vi "SetInstrument type.vi"(0 "object in":refnum<class "KE2410.lvclass">, 1 "Instrument type":enum16{""}(ring), 5 "error in (no error)":errorcluster) -> (14 "object out":refnum<class "KE2410.lvclass">, 19 "error out":errorcluster)   [LabVIEW 2013, in "KE2410.lvclass"]
uses:
  KE2410.lvclass
  KE2410.lvclass/KE2410.ctl
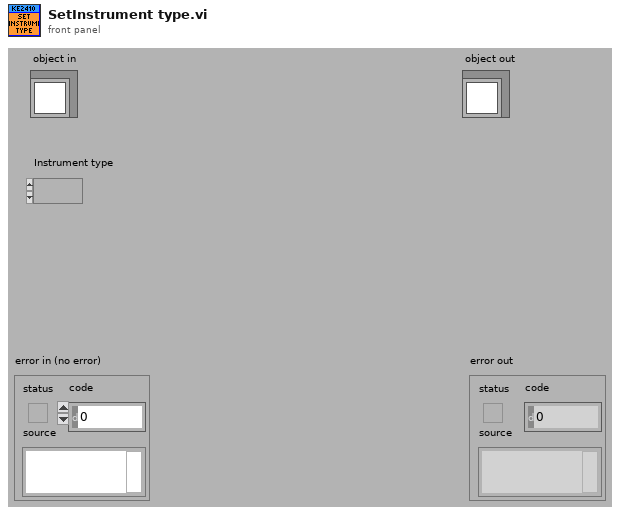
[diagram p1: front panel]
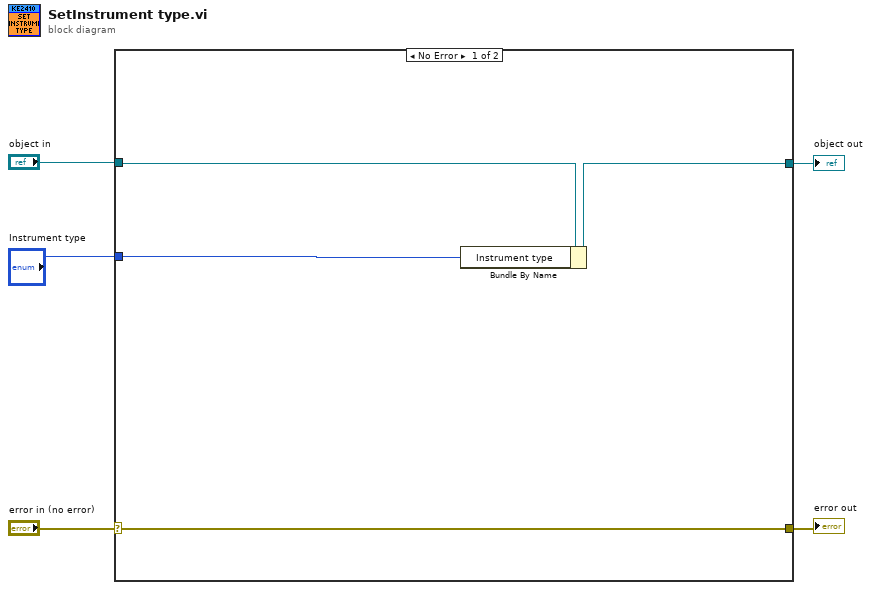
[diagram p0: block diagram]
diagram:
  n1 = case shown="No Error" "error in (no error)" {
    selector: "error in (no error)" -> [w8 w11]
    tunnel: [w8 w11] -> w4
    tunnel: [w6 w10] -> w2
    tunnel: "object in" -> [w7 w10]
    tunnel: "Instrument type" -> [w9 _]
    frame No Error {
      n2 = Bundle By Name(cluster=w7, "Instrument type"=w9) -> (w6:refnum<class "KE2410.lvclass">)
    }
    frame Error {
    }
  }
  "error out" <- w4
  "object out" <- w2
